vi "ContourBasedSegement.vi"() -> ()   [LabVIEW 2016]
doc: "This example shows how to use the Edge Tool in NI Vision. The Edge Tool finds edges (or sharp transitions in the pixels values) along a given line or ROI profile. The Edge Tool is a precursor function to many of the gauging and inspection tasks. For example, the location of the edges found along a line profile across an object can interpreted as the boundaries of the object whose dimensions have to be measured for a gauging application or the presence of a crack in the surface of an object for an inspection application."
uses:
  <vilib>/vision/Contour.llb/IMAQ Contour Curve Extraction.ctl
  <vilib>/vision/Contour.llb/IMAQ Connect Range Setting.ctl
  <vilib>/vision/NI_Vision_Development_Module.lvlib
panel:
  in  "Contour Selection":T1(ring)
  in  "Search Direction":T2(ring)
  in  "Curve Connection":T3[](array[typedef])=[{"Match Constraints"=0, "Min"=0.0, "Max"=25.0}, {"Match Constraints"=1, "Min"=0.0, "Max"=180.0}, {"Match Constraints"=2, "Min"=0.0, "Max"=25.0}, {"Match Constraints"=3, "Min"=0.0, "Max"=180.0}] {"Max" format="%.2f"; "Min" format="%.2f"; "Match Constraints" items=["Distance (pixel)", "Angle Difference (degrees)", "Connectivity Distance (pixel)", "Gradient Difference (degrees)"]}
  in  "Curve Extraction":T4={"Extraction Mode"=0, "Edge Threshold"=128, "Edge Filter Size"=2, "Min Length"=25, "Search Step Size"=10, "Max Endpoint Gap"=10, "Subpixel"=TRUE} {"Extraction Mode" items=["Normal", "Uniform Regions"]; "Edge Filter Size" items=["Fine", "Normal", "Contour Tracing"]; "Max Endpoint Gap" min=0; "Search Step Size" min=1 max=255 step=1; "Min Length" min=0; "Edge Threshold" min=1 max=350 step=1}
  out "Image":T5(plugin-control)
  in  "Stop":bool
  # "Range"
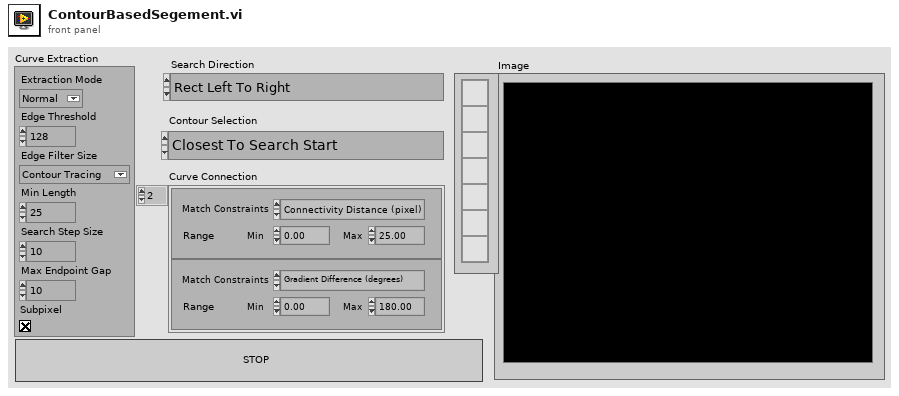
[diagram p1: front panel]
types:
  T1 = enum16{"Closest To Search Start", "Maximum Length", "Strongest Mean Gradient Change"}
  T2 = enum16{"Rect Left To Right", "Rect Right To Left", "Rect Top To Bottom", "Rect Bottom To Top", "Annulus Inner To Outer", "Annulus Outer To Inner", "Annulus Start Angle To End Angle", "Annulus End Angle To Start Angle"}
  T3 = typedef "IMAQ Connect Range Setting.ctl" = cluster{"Match Constraints":u32, "Min":dbl, "Max":dbl}
  T4 = typedef "IMAQ Contour Curve Extraction.ctl" = cluster{"Extraction Mode":u32, "Edge Threshold":i32, "Edge Filter Size":u32, "Min Length":i32, "Search Step Size":i32, "Max Endpoint Gap":i32, "Subpixel":bool}
  T5 = typedef "IMAQ Image.ctl" = refnum<image>
  T6 = typedef "IMAQ Rectangle" = cluster{"Left":i32, "Top":i32, "Right":i32, "Bottom":i32, "Rotation":dbl}
  T7 = typedef "ROI Descriptor" = cluster{"Global Rectangle":i32[], "Contours":cluster{"ID":enum32{"External", "Internal"}, "Type":u32, "Coordinates":i32[]}[]}
  T8 = cluster{"Curve Extraction":T4, "Curve Connection":T3[], "Search Direction":enum16{"Rect Left To Right", "Rect Right To Left", "Rect Top To Bottom", "Rect Bottom To Top", "Annulus Inner To Outer", "Annulus Outer To Inner", "Annulus Start Angle To End Angle", "Annulus End Angle To Start Angle"}, "Contour Selection":enum16{"Closest To Search Start", "Maximum Length", "Strongest Mean Gradient Change"}}
  T9 = cluster{"Overlay?":bool, "Color":u32, "Width":u32, "Maintain Width?":bool}
  T10 = cluster{"Global Rectangle":i32[], "Contours":cluster{"Contour Type":u32, "ROI Type":u32, "Points":i32[]}[]}
  T11 = cluster{"Global Rectangle":i32[], "Contours":cluster{"ID":enum32{"External", "Internal"}, "Type":u32, "Coordinates":i32[]}[]}
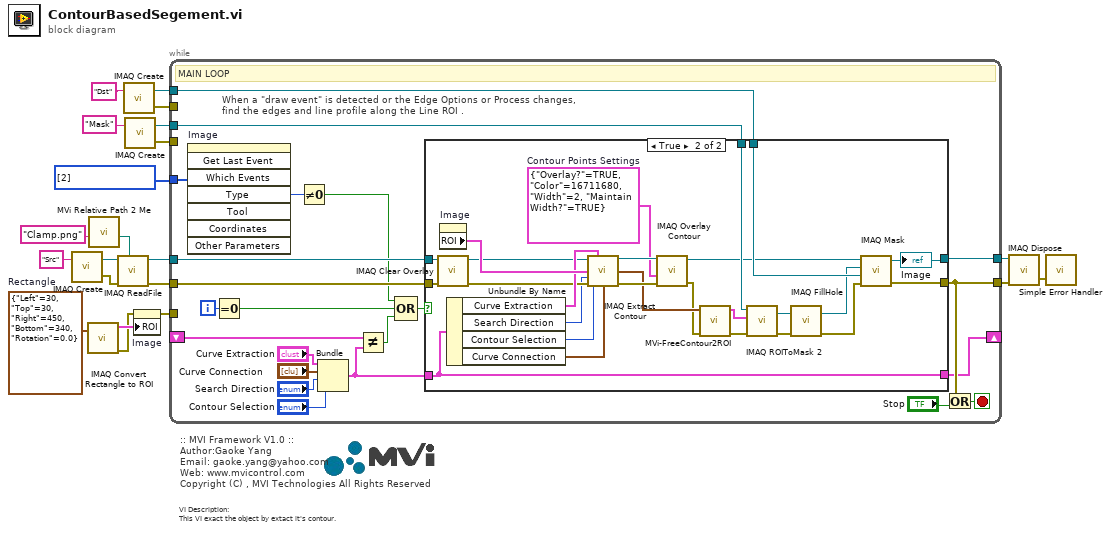
[diagram p0: block diagram]
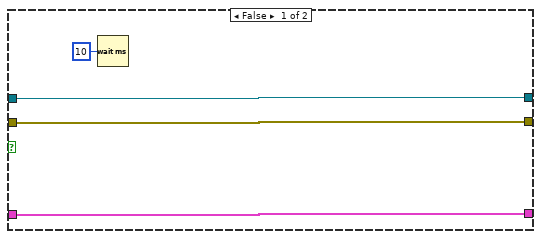
[diagram p2: hidden frame]
diagram:
  w9 = T6 {"Left"=30, "Top"=30, "Right"=450, "Bottom"=340, "Rotation"=0.0}  # Rectangle
  w14 = i32[] [2] items=["No  event", "Click event", "Draw event", "Move event", "Size event", "Scroll event", "Activate event", "Close event", "Double click event"] ("Events list (all)")
  # "VI Description:\nThis VI exact the object by extact it's contour."
  # ":: MVI Framework V1.0 ::\nAuthor:Gaoke Yang\nEmail: gaoke.yang@yahoo.com\nWeb: www.mvicontrol.com\nCopyright (C) , MVI Technologies All Rights Reserved"
  n1 = call "IMAQ Create"("Image Name"="Src") -> ("New Image"=w20:T5, "error out"=w19:errorcluster)  [unwired: 4 in]
  n2 = call "IMAQ Convert Rectangle to ROI"("Rectangle"=w9) -> ("error out"=w8:errorcluster, "ROI Descriptor"=w11:T7)  [unwired: 8 in]
  n3 = call "MVi Relative Path 2 Me.vi"("Relative Path"="Clamp.png" ("name or relative path")) -> ("Appended Dir"=w12:path)  [unwired: 5 in, 1 out]
  n4 = call "IMAQ ReadFile"("File Path"=w12, "error in (no error)"=w19, "Image"=w20) -> ("error out"=w15:errorcluster, "Image Out"=w16:T5)  [unwired: 4 in, 3 out]
  n5 = call "IMAQ Create"("Image Name"="Dst") -> ("New Image"=w3:T5, "error out"=w1:errorcluster)  [unwired: 4 in]
  n6 = call "IMAQ Create"("Image Name"="Mask") -> ("New Image"=w4:T5, "error out"=w2:errorcluster)  [unwired: 4 in]
  n7 = property on="Image" class="ImageControl"(error in=w8, "ROI"=w11) -> (error out=w10:errorcluster)  [unwired: 1 in, 1 out]
  n8 = while "MAIN LOOP" {
    tunnel: w16 -> [w42]
    tunnel: w15 -> [w43]
    tunnel: [w38] -> w18
    tunnel: [w39] -> w17
    tunnel: w14 -> [w37]
    shift-right: [w32] -> _
    shift-left: _ -> [w29]
    tunnel: w10 -> [_]
    tunnel: w4 -> [w23]
    tunnel: w3 -> [w22]
    tunnel: w2 -> [_]
    tunnel: w1 -> [_]
    i -> [w35]
    stop <- w40 stop-if-true
    # "When a \"draw event\" is detected or the Edge Options or Process changes, find the edges and line profile along the Line ROI ."
    # "MAIN LOOP"
    n9 = invoke on="Image" class="ImageControl" method="Get Last Event"("Which Events"=w37) -> ("Type"=w36:i32)  [unwired: 7 in, 7 out]
    n10 = Equal To 0?(x=w35) -> (x = 0?=w31:bool)
    n11 = Not Equal To 0?(x=w36) -> (x != 0?=w34:bool)
    n12 = Bundle("Curve Extraction"="Curve Extraction", "Curve Connection"="Curve Connection", "Search Direction"="Search Direction", "Contour Selection"="Contour Selection") -> (w30:T8)  [unwired: 1 in]
    n13 = Not Equal?(x=w29, y=w30) -> (x != y?=w28:bool)
    n14 = Compound Arithmetic op=OR(w34, w31, w28) -> (w33:bool)
    n15 = case shown="True" w33 {
      tunnel: w43 -> [w46 w73]
      tunnel: w42 -> [w47 w72]
      tunnel: [w47 w48] -> w39
      tunnel: [w46 w57] -> w38
      tunnel: [w44 w71] -> w32
      tunnel: w30 -> [w44 w71]
      tunnel: w23 -> [_ w56]
      tunnel: w22 -> [_ w55]
      frame False {
        n16 = Wait (ms)(milliseconds to wait=u32 10) -> ()  [unwired: 1 out]
      }
      frame True {
        w61 = T9 {"Overlay?"=TRUE, "Color"=16711680, "Width"=2, "Maintain Width?"=TRUE}  # Contour Points Settings
        n17 = call "IMAQ Clear Overlay"("error in (no error)"=w73, "Image"=w72) -> ("error out"=w68:errorcluster, "Image Out"=w64:T5)  [unwired: 8 in]
        n18 = property on="Image" class="ImageControl"() -> ("ROI"=w70:T10)  [unwired: 2 in, 2 out]
        n19 = Unbundle By Name(w71) -> ("Curve Extraction"=w69:T4, "Search Direction"=w67:T2, "Contour Selection"=w66:T1, "Curve Connection"=w65:T3[])
        n20 = call "IMAQ Extract Contour"("Source Image"=w64, "Curve Extraction"=w69, "ROI Descriptor"=w70, "Search Direction"=w67, "error in (no error)"=w68, "Contour Selection"=w66, "Curve Connection"=w65) -> ("Source Image Out"=w62:T5, "Contour Points"=w60:cluster{"X":dbl, "Y":dbl}[], "error out"=w63:errorcluster)  [unwired: 4 in, 2 out]
        n21 = call "IMAQ Overlay Contour"("error in (no error)"=w63, "Contour Points Settings"=w61, "Image"=w62) -> ("error out"=w59:errorcluster, "Image Out"=w50:T5)  [unwired: 3 in, 4 out]
        n22 = call "MVi-FreeContour2ROI.vi"("ErrIn"=w59, "Contour\nPoints"=w60) -> ("ErrOut"=w58:errorcluster, "ROI\nDescriptor"=w54:T11)  [unwired: 8 in]
        n23 = call "IMAQ ROIToMask 2"("error in (no error)"=w58, "ROI Descriptor"=w54, "Image"=w56) -> ("error out"=w52:errorcluster, "Image Out"=w53:T5)  [unwired: 6 in, 1 out]
        n24 = call "IMAQ FillHole"("error in (no error)"=w52, "Image Src"=w53) -> ("error out"=w51:errorcluster, "Image Dst Out"=w49:T5)  [unwired: 4 in]
        n25 = call "IMAQ Mask"("error in (no error)"=w51, "Image Dst"=w55, "Image Mask"=w49, "Image Src"=w50) -> ("error out"=w57:errorcluster, "Image Dst Out"=w48:T5)  [unwired: 1 in]
        "Image" <- w48
      }
    }
    n26 = Or(x=w38, y="Stop") -> (x .or. y?=w40:bool)
  }
  n27 = call "IMAQ Dispose"("Image"=w17, "error in (no error)"=w18) -> ("error out"=w7:errorcluster)  [unwired: 4 in]
  n28 = call <vilib>:"Simple Error Handler.vi"("error in (no error)"=w7) -> ()  [unwired: 4 in, 5 out]
